vi "OnDataChange.vi"(0 "Prime95BCameraController in":refnum<class "CameraController.lvclass">, 1 "DataExchange":T1, 3 "error in (no error)":errorcluster) -> (7 "Prime95BCameraController out":refnum<class "CameraController.lvclass">, 10 "error out":errorcluster)   [LabVIEW 2020, in "CameraController.lvlib" / "CameraController.lvclass"]
uses:
  CameraController.lvclass
  Model/Hardware Abstraction Layer/Component/Device/Device/DataExchange.ctl
  Interface/DataListener/DataListener.lvclass
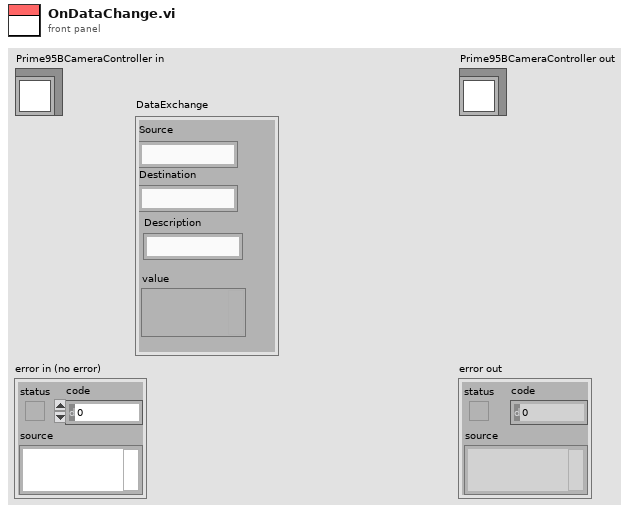
[diagram p1: front panel]
types:
  T1 = typedef "DataListener.lvclass/DataExchange.ctl" = cluster{"Source":string, "Destination":string, "Description":string, "value":variant}
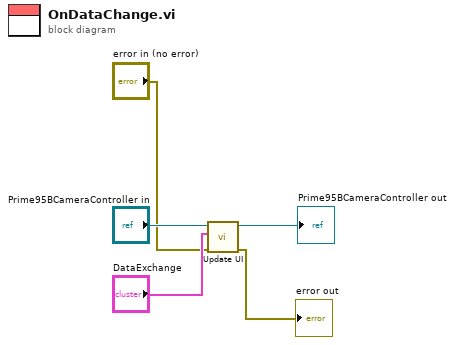
[diagram p0: block diagram]
diagram:
  n1 = call-dynamic "Update UI.vi"("error in (no error)"="error in (no error)", "DataExchange"="DataExchange", "Camera Prime95B Controller in"="Prime95BCameraController in") -> ("error out"=→"error out":errorcluster, "Camera Prime95B Controller out"=→"Prime95BCameraController out":refnum<class "CameraController.lvclass">)  [unwired: 7 in]
